vi "Var_Write_Sim.vi"   [LabVIEW 2021]
uses:
  Support/DBL/Var_DBL.lvclass
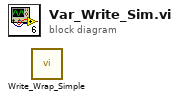
[diagram p0: block diagram]
diagram:
  n1 = call "Write_Wrap_Simple.vi"() -> ()  [unwired: 5 in, 1 out]
